vi "getCheckSum.vi"(8 "error in (no error)":errorcluster, 10 "response":string=".0101WatchDog", 11 "CoolerSerialCommand in":refnum<class "CoolerSerialCommand.lvclass">) -> (0 "error out":errorcluster, 2 "Checksum":string, 3 "CoolerSerialCommand out":refnum<class "CoolerSerialCommand.lvclass">)   [LabVIEW 2016, in "CoolerSerialCommand.lvclass"]
uses:
  CoolerSerialCommand.lvclass
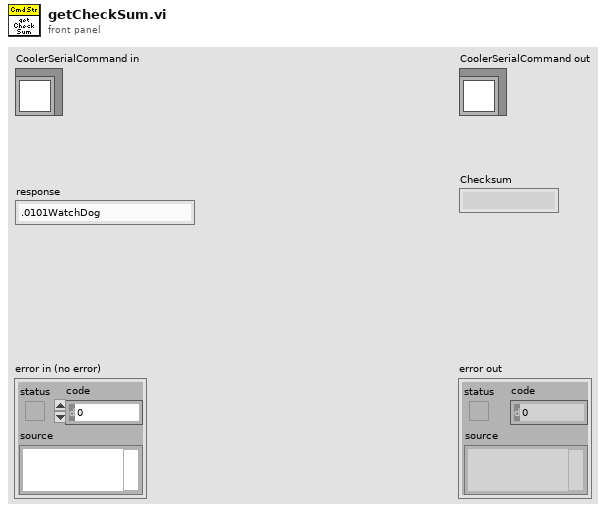
[diagram p1: front panel]
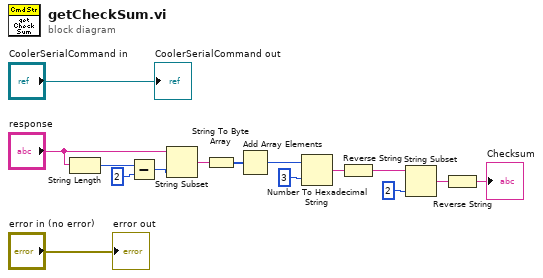
[diagram p0: block diagram]
diagram:
  n1 = String Length(string="response") -> (length=w3:i32)
  n2 = Subtract(x=w3, y=2) -> (x-y=w1:i32)
  n3 = String Subset(string="response", length (rest)=w1) -> (substring=w5:string)  [unwired: 1 in]
  n4 = String To Byte Array(string=w5) -> (unsigned byte array=w7:u8[])
  n5 = Add Array Elements(numeric array=w7) -> (sum=w13:u8)
  n6 = Number To Hexadecimal String(1:i16 3 ("width (-)"), 2:w13) -> (0:w11:string)
  n7 = Reverse String(1:w11) -> (0:w10:string)
  n8 = String Subset(string=w10, length (rest)=2 ("length (rest)")) -> (substring=w9:string)  [unwired: 1 in]
  n9 = Reverse String(1:w9) -> (0:→"Checksum":string)
  "error out" <- "error in (no error)"
  "CoolerSerialCommand out" <- "CoolerSerialCommand in"
